vi "Reset.vi"(7 "Micropulse # In":i32, 8 "error in (no error)":errorcluster, 9 "Hard Reset?":bool caption="Hard Reset? (def: F - Soft Reset)", 10 "Sample Frequency":T1) -> (0 "error out":errorcluster, 2 "Micropulse Settings Out":T2={"Instrument Type"=enum."MicroPulse 5", "Serial #"=0, "Sample Frequency"=enum."100MHz", "dt (us)"=0.0, "DOF"=enum."", "Material Velocity"=1.0, "Asynch Reads"=enum."Disabled", "NUM of Tests"=0, "System Details"={"System Type"=enum."MicroPulse 5", "Serial No."=0, "Channels"={"Conv"=0, "PA"=0, "Extra"=0}, "Sample Frequency"={"Default"=0, "Actual"=0}, "Software Versions"="", "Data Output Format"={"Default"=enum."8-bit Mode", "Actual"=enum."8-bit Mode"}, "Temperatures"={"System"=0, "Processor"=0, "Slave Sys"=0, "Slave Proc"=0}, "Tx Buffer Size"=0, "System Error"="", "No. of Cards"=0, "DAC Gain"=0, "Uptimes"={"since Power"=0, "since RSTS"=0, "since SRST"=0}, "Voltages"=[], "Interface Cards"=[]}, "Gates"=[], "Encoders"=[], "CMD LUT"=variant, "Command List"=""} {"System Details"."Interface Cards"."FPGA - T" format="%.0f °C"; "System Details"."Interface Cards"."Board - T" format="%.0f °C"; "System Details"."Voltages"."Difference" format="%.2fV"; "System Details"."Voltages"."Measured" format="%.2fV"; "System Details"."Voltages"."Nominal" format="%.2fV"; "System Details"."DAC Gain" format="%.0fdB"; "System Details"."Tx Buffer Size" format="%.0fMB"; "System Details"."Temperatures"."Slave Proc" format="%.0f C"; "System Details"."Temperatures"."Slave Sys" format="%.0f C"; "System Details"."Temperatures"."Processor" format="%.0f C"; "System Details"."Temperatures"."System" format="%.0f C"; "System Details"."Sample Frequency"."Actual" format="%.0fMHz"; "System Details"."Sample Frequency"."Default" format="%.0fMHz"; "Encoders"."Encoder Filter" max=255; "Encoders"."Backlash Period (s)" min=0.0005 max=10.0 step=0.0005; "Encoders"."Multiplier" min=1 max=100000; "Encoders"."Counts/mm" min=1 max=100000; "Gates"."Insp Gates"."Max # Peaks" max=64000 step=100; "Gates"."Insp Gates"."Threshold" min=10 max=4095 step=10; "Gates"."Insp Gates"."Length (us)" min=0.0 max=96000.0 step=100.0; "Gates"."Insp Gates"."Start (us)" min=0.0 max=64000.0 step=100.0; "Gates"."Echo Gate"."Threshold" min=10 max=4095 step=10; "Gates"."Echo Gate"."Length (us)" min=0.0 max=96000.0 step=100.0; "Gates"."Echo Gate"."Start (us)" min=0.0 max=64000.0 step=100.0; "Gates"."Display Gate"."Length" min=0.0 max=64000.0 step=1000.0; "Gates"."Display Gate"."Start" min=0.0 max=64000.0 step=1000.0}, 5 "Micropulse # Out":i32)   [LabVIEW 2015, in "MicroPulse_Driver.lvlib"]
doc: "Performs either a hard or a soft reset of the Micropulse instrument depending on the value of <b>Hard Reset?</b>\nReturns the instrument to its power on state.\nOptionally allows for changing the sampling rate from the instrument's default.\nReturns the new settings data in <b>Micropulse Settings Out</b>."
uses:
  <instrlib>/MicroPulse/MicroPulse_Driver.lvlib
  <instrlib>/MicroPulse/Public/Data/Datatypes/MP-Registry Data-Cluster.ctl
  <instrlib>/MicroPulse/Public/Data/Datatypes/MP - instrument type.ctl
  <instrlib>/MicroPulse/Public/Data/Datatypes/MP - sample frequency.ctl
  <instrlib>/MicroPulse/Public/Data/Datatypes/MP - data output format.ctl
  <instrlib>/MicroPulse/Public/Data/Datatypes/MP - asynch read mode.ctl
  <instrlib>/MicroPulse/Public/Data/Datatypes/MP - general system status.ctl
  <instrlib>/MicroPulse/Public/Data/Datatypes/MP - interface card status.ctl
  <instrlib>/MicroPulse/Public/Data/Datatypes/subdatatypes/MP - Registry Gates.ctl
  <instrlib>/MicroPulse/Public/Data/Datatypes/MP - display gate.ctl
  <instrlib>/MicroPulse/Public/Data/Datatypes/MP - echo gate mode.ctl
  <instrlib>/MicroPulse/Public/Data/Datatypes/MP - echo gate parameters.ctl
  <instrlib>/MicroPulse/Public/Data/Datatypes/MP - multigate inspection gate parameters.ctl
  <instrlib>/MicroPulse/Public/Data/Datatypes/MP - hysteresis level.ctl
  <instrlib>/MicroPulse/Public/Data/Datatypes/MP - multigate mode.ctl
  <instrlib>/MicroPulse/Public/Data/Datatypes/MP - encoder settings.ctl
  <instrlib>/MicroPulse/Public/Data/Datatypes/MP - encoder type.ctl
  <instrlib>/MicroPulse/Private/MP-Registry Action-Enum.ctl
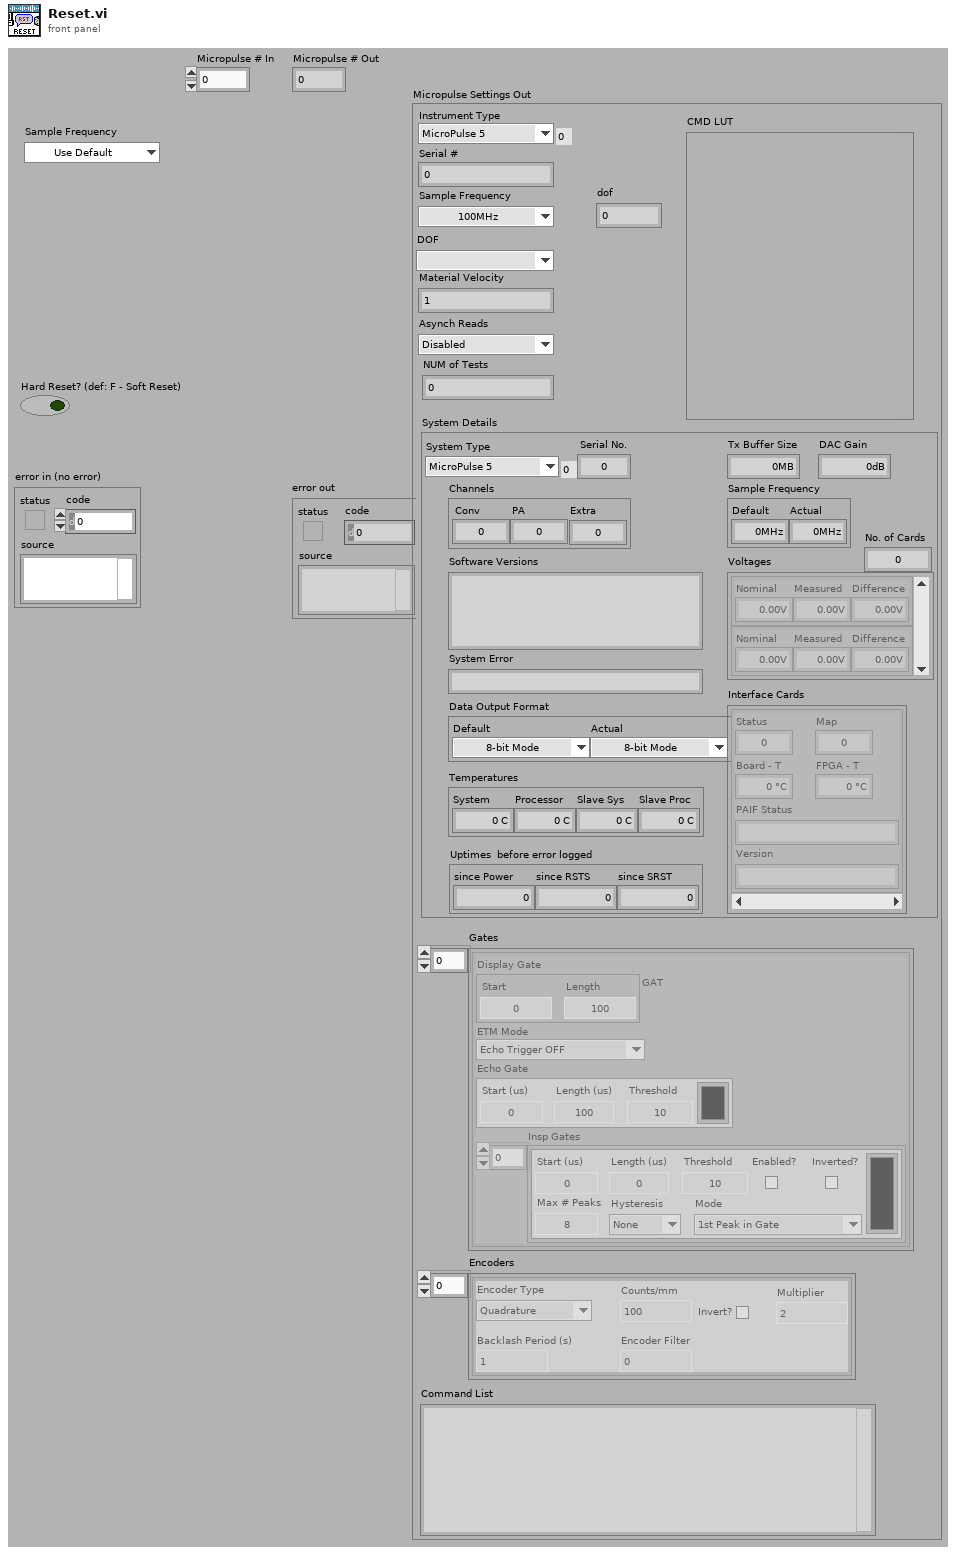
[diagram p1: front panel]
types:
  T1 = typedef "MicroPulse_Driver.lvlib/MP - sample frequency.ctl" = enum16{"Use Default", "200MHz (LT2 only)", "100MHz", "50MHz", "25MHz", "10MHz"}
  T2 = typedef "MicroPulse_Driver.lvlib/MP-Registry Data-Cluster.ctl" = cluster{"Instrument Type":T3, "Serial #":u64, "Sample Frequency":T1, "dt (us)":dbl, "DOF":T4, "Material Velocity":dbl, "Asynch Reads":T5, "NUM of Tests":u32, "System Details":T6, "Gates":T8[], "Encoders":T15[], "CMD LUT":variant, "Command List":string}
  T3 = typedef "MicroPulse_Driver.lvlib/MP - instrument type.ctl" = enum16{"MicroPulse 5", "LT1", "LT2", "LTPA", "MPLT", "MicroPulse 6", "<MicroPulse>", "Micropulse 4", "Simulated Data"}
  T4 = typedef "MicroPulse_Driver.lvlib/MP - data output format.ctl" = enum16{"", "8-bit Mode", "10-bit Mode", "12-bit Mode", "16-bit Mode", "8-bit Log Mode", "12-bit Packed Mode"}
  T5 = typedef "MicroPulse_Driver.lvlib/MP - asynch read mode.ctl" = enum16{"Disabled", "Enabled"}
  T6 = typedef "MicroPulse_Driver.lvlib/MP - general system status.ctl" = cluster{"System Type":T3, "Serial No.":u64, "Channels":cluster{"Conv":u8, "PA":u16, "Extra":u32}, "Sample Frequency":cluster{"Default":u8, "Actual":u8}, "Software Versions":string, "Data Output Format":cluster{"Default":T4, "Actual":T4}, "Temperatures":cluster{"System":u8, "Processor":u8, "Slave Sys":u8, "Slave Proc":u8}, "Tx Buffer Size":u32, "System Error":string, "No. of Cards":u8, "DAC Gain":i16, "Uptimes":cluster{"since Power":u32, "since RSTS":u32, "since SRST":u32}, "Voltages":cluster{"Nominal":dbl, "Measured":dbl, "Difference":dbl}[], "Interface Cards":T7[]}
  T7 = typedef "MicroPulse_Driver.lvlib/MP - interface card status.ctl" = cluster{"Status":u8, "Map":u8, "Board - T":u8, "FPGA - T":u8, "PAIF Status":string, "Version":string}
  T8 = typedef "MicroPulse_Driver.lvlib/MP - Registry Gates.ctl" = cluster{"Display Gate":T9, "ETM Mode":T10, "Echo Gate":T11, "Insp Gates":T12[]}
  T9 = typedef "MicroPulse_Driver.lvlib/MP - display gate.ctl" = cluster{"Start":dbl, "Length":dbl}
  T10 = typedef "MicroPulse_Driver.lvlib/MP - echo gate mode.ctl" = enum16{"Echo Trigger OFF", "Echo Gate Display Mode", "Echo Trigger ON", "Multi Gate or FMC Mode", "Reserved", "PA - Echo Trigger ON"}
  T11 = typedef "MicroPulse_Driver.lvlib/MP - echo gate parameters.ctl" = cluster{"Start (us)":dbl, "Length (us)":dbl, "Threshold":u16, "Colour":u32}
  T12 = typedef "MicroPulse_Driver.lvlib/MP - multigate inspection gate parameters.ctl" = cluster{"Start (us)":dbl, "Length (us)":dbl, "Threshold":u16, "Enabled?":bool, "Max # Peaks":u16, "Hysteresis":T13, "Mode":T14, "Inverted?":bool, "Colour ":u32}
  T13 = typedef "MicroPulse_Driver.lvlib/MP - hysteresis level.ctl" = enum16{"None", "3dB", "6dB", "9dB", "12dB"}
  T14 = typedef "MicroPulse_Driver.lvlib/MP - multigate mode.ctl" = enum16{"1st Peak in Gate", "Largest Peak In Gate", "All Peaks In Gate", "1st Threshold Crossing"}
  T15 = typedef "MicroPulse_Driver.lvlib/MP - encoder settings.ctl" = cluster{"Encoder Type":T16, "Counts/mm":u32, "Invert?":bool, "Multiplier":u32, "Backlash Period (s)":dbl, "Encoder Filter":u32}
  T16 = typedef "MicroPulse_Driver.lvlib/MP - encoder type.ctl" = enum16{"Quadrature", "Step/Direction"}
  T17 = typedef "MicroPulse_Driver.lvlib/MP-Registry Action-Enum.ctl" = enum16{"Read", "Add Test", "Add Command", "Add Gate Command", "Add Encoder Command", "Clear Command  List", "Set Registry", "Set System Details", "Set DOF", "Set Velocity", "Disable Asynch Reads", "Enable Asynch Reads", "Add Connection", "Disconnect", "Shutdown"}
  T18 = typedef "MicroPulse_Driver.lvlib/TCP config.ctl" = cluster{"Connection ID":refnum<k5>, "IP address":string, "host port":u16, "OC timeout":i32, "Read timeout":i32, "Write timeout":i32}
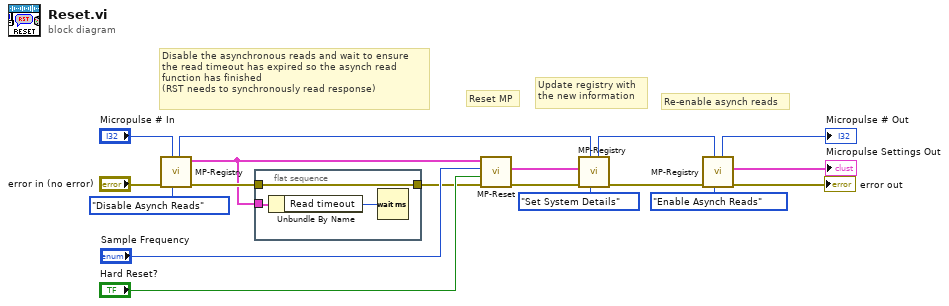
[diagram p0: block diagram]
diagram:
  # "Update registry with\nthe new information"
  # "Re-enable asynch reads"
  # "Reset MP"
  # "Disable the asynchronous reads and wait to ensure\nthe read timeout has expired so the asynch read\nfunction has finished\n(RST needs to synchronously read response)"
  n1 = call <instrlib>:"MP-Registry.vi"("Action"=MP-Registry_Action-Enum."Disable Asynch Reads", "Micropulse # In"="Micropulse # In", "error in (no error)"="error in (no error)") -> ("error out"=w3:errorcluster, "TCP config"=w1:T18, "Micropulse # Out"=w12:i32)  [unwired: 5 in, 1 out]
  n2 = flat-sequence {
    tunnel: w1 -> [w20]
    tunnel: w3 -> [w21]
    tunnel: [w21] -> w2
    frame #0 {
      n3 = Unbundle By Name(w20) -> ("Read timeout"=w19:i32)
      n4 = Wait (ms)(milliseconds to wait=w19) -> ()  [unwired: 1 out]
    }
  }
  n5 = call <instrlib>:"MP-Reset.vi"("error in (no error)"=w2, "Hard Reset?"="Hard Reset?", "Sample Frequency"="Sample Frequency", "TCP config"=w1) -> ("error out"=w14:errorcluster, "System Status"=w13:T6)  [unwired: 5 in, 1 out]
  n6 = call <instrlib>:"MP-Registry.vi"("Action"=MP-Registry_Action-Enum."Set System Details", "Micropulse # In"=w12, "error in (no error)"=w14, "Data in"=w13) -> ("error out"=w8:errorcluster, "Micropulse # Out"=w6:i32)  [unwired: 4 in, 2 out]
  n7 = call <instrlib>:"MP-Registry.vi"("Action"=MP-Registry_Action-Enum."Enable Asynch Reads", "Micropulse # In"=w6, "error in (no error)"=w8) -> ("error out"=→"error out":errorcluster, "Micropulse Data"=→"Micropulse Settings Out":T2, "Micropulse # Out"=→"Micropulse # Out":i32)  [unwired: 5 in, 1 out]
